vi "写入内置参数.vi"(7 "量程参数读取":T3 {"阈值（高->低）" format="%#.6g"; "阈值（低->高）" format="%#.6g"; "下限" format="%#.6g"; "上限" format="%#.6g"}, 8 "error in (no error)":errorcluster, 9 "float":T2 {"偏心轮校准参数" format="%#.6g"}, 10 "外设配置":T1 {"是否存在液位检测板" items=["否", "是"]; "阀数量" items=["9通"=9, "12通"=12]; "泵类型" items=["TECAN", "润泽"]}, 11 "MB session in":refnum<class "MB_Master.lvclass">) -> (0 "error out":errorcluster, 3 "MB session out":refnum<class "MB_Master.lvclass">)   [LabVIEW 2016, in "斯坦道CODMn新电路板.lvlib"]
uses:
  <vilib>/Plasmionique/MB Master/MB_Master/MB_Master.lvclass
  <vilib>/Plasmionique/MB Master/MB_Master_Serial/MB_Master_Serial.lvclass
  D:/Program Files (x86)/National Instruments/LabVIEW 2016/vi.lib/Plasmionique/MB Master/MB_Master/MB_Master.lvclass
  <vilib>/Plasmionique/MB Master/MB Master.lvlib
panel:
  in  "VISA Resource":refnum<visa-resource-name>
  in  "引用选择":enum16{"MB引用", "自建引用"}(ring)
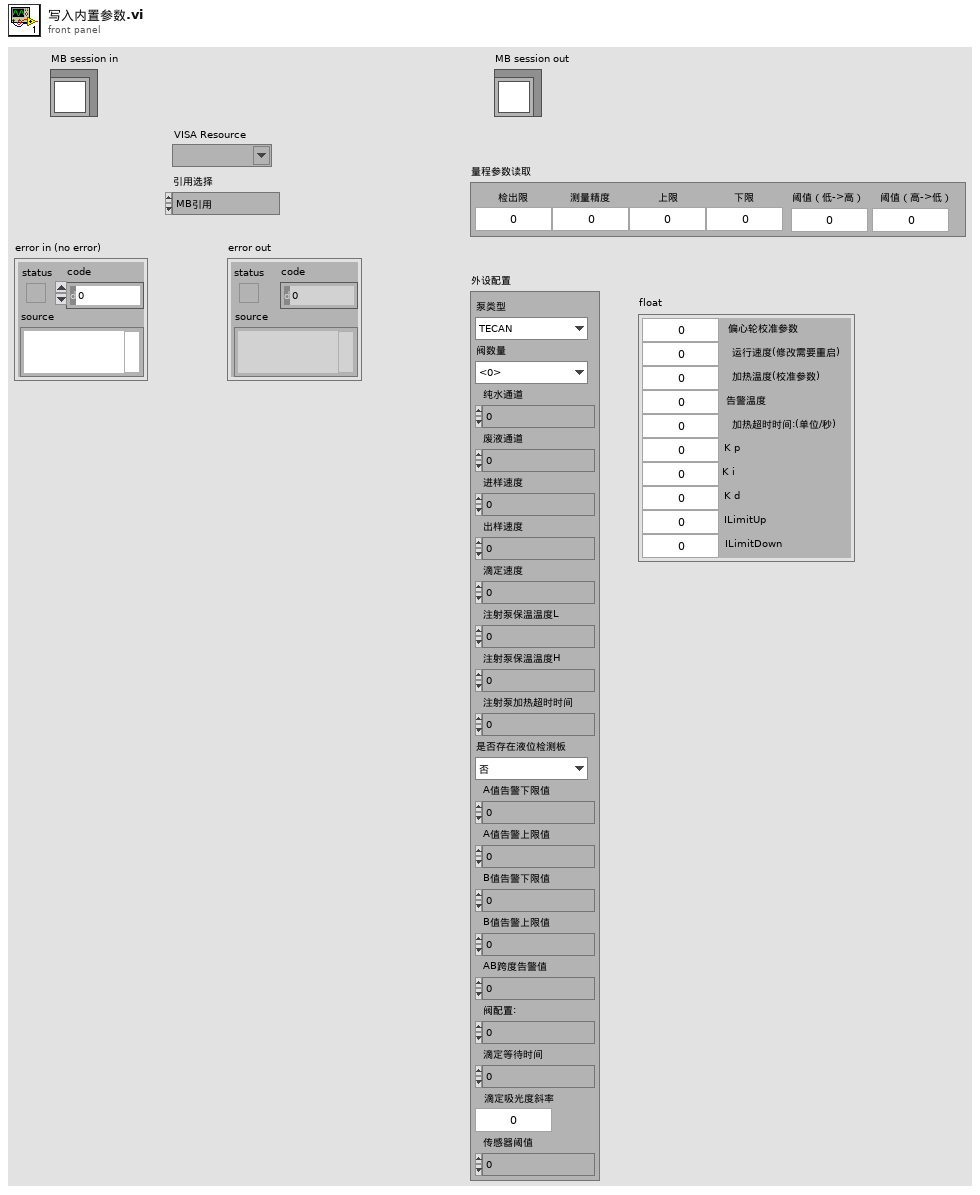
[diagram p1: front panel]
types:
  T1 = cluster{"泵类型":u8, "阀数量":u8, "纯水通道":u16, "废液通道":u8, "进样速度":u16, "出样速度":u16, "滴定速度":u16, "注射泵保温温度L":u8, "注射泵保温温度H":u8, "注射泵加热超时时间":u16, "是否存在液位检测板":u16, "A值告警下限值":u16, "A值告警上限值":u16, "B值告警下限值":u16, "B值告警上限值":u16, "AB跨度告警值":u16, "阀配置:":u8, "滴定等待时间":u16, "滴定吸光度斜率":dbl, "传感器阈值":u16}
  T2 = cluster{"偏心轮校准参数":dbl, "运行速度(修改需要重启)":u16, "加热温度(校准参数) ":dbl, "告警温度":dbl, "加热超时时间:(单位/秒)":dbl, "K p":dbl, "K i":dbl, "K d":dbl, "ILimitUp":dbl, "ILimitDown":dbl}
  T3 = cluster{"检出限":dbl, "测量精度":dbl, "上限":dbl, "下限":dbl, "阈值（低->高）":dbl, "阈值（高->低）":dbl}
  T4 = cluster{"baud rate (bps)":u32, "stop bits":u16, "parity":u16, "flow control":u16, "timeout":u32, "retries":i32}
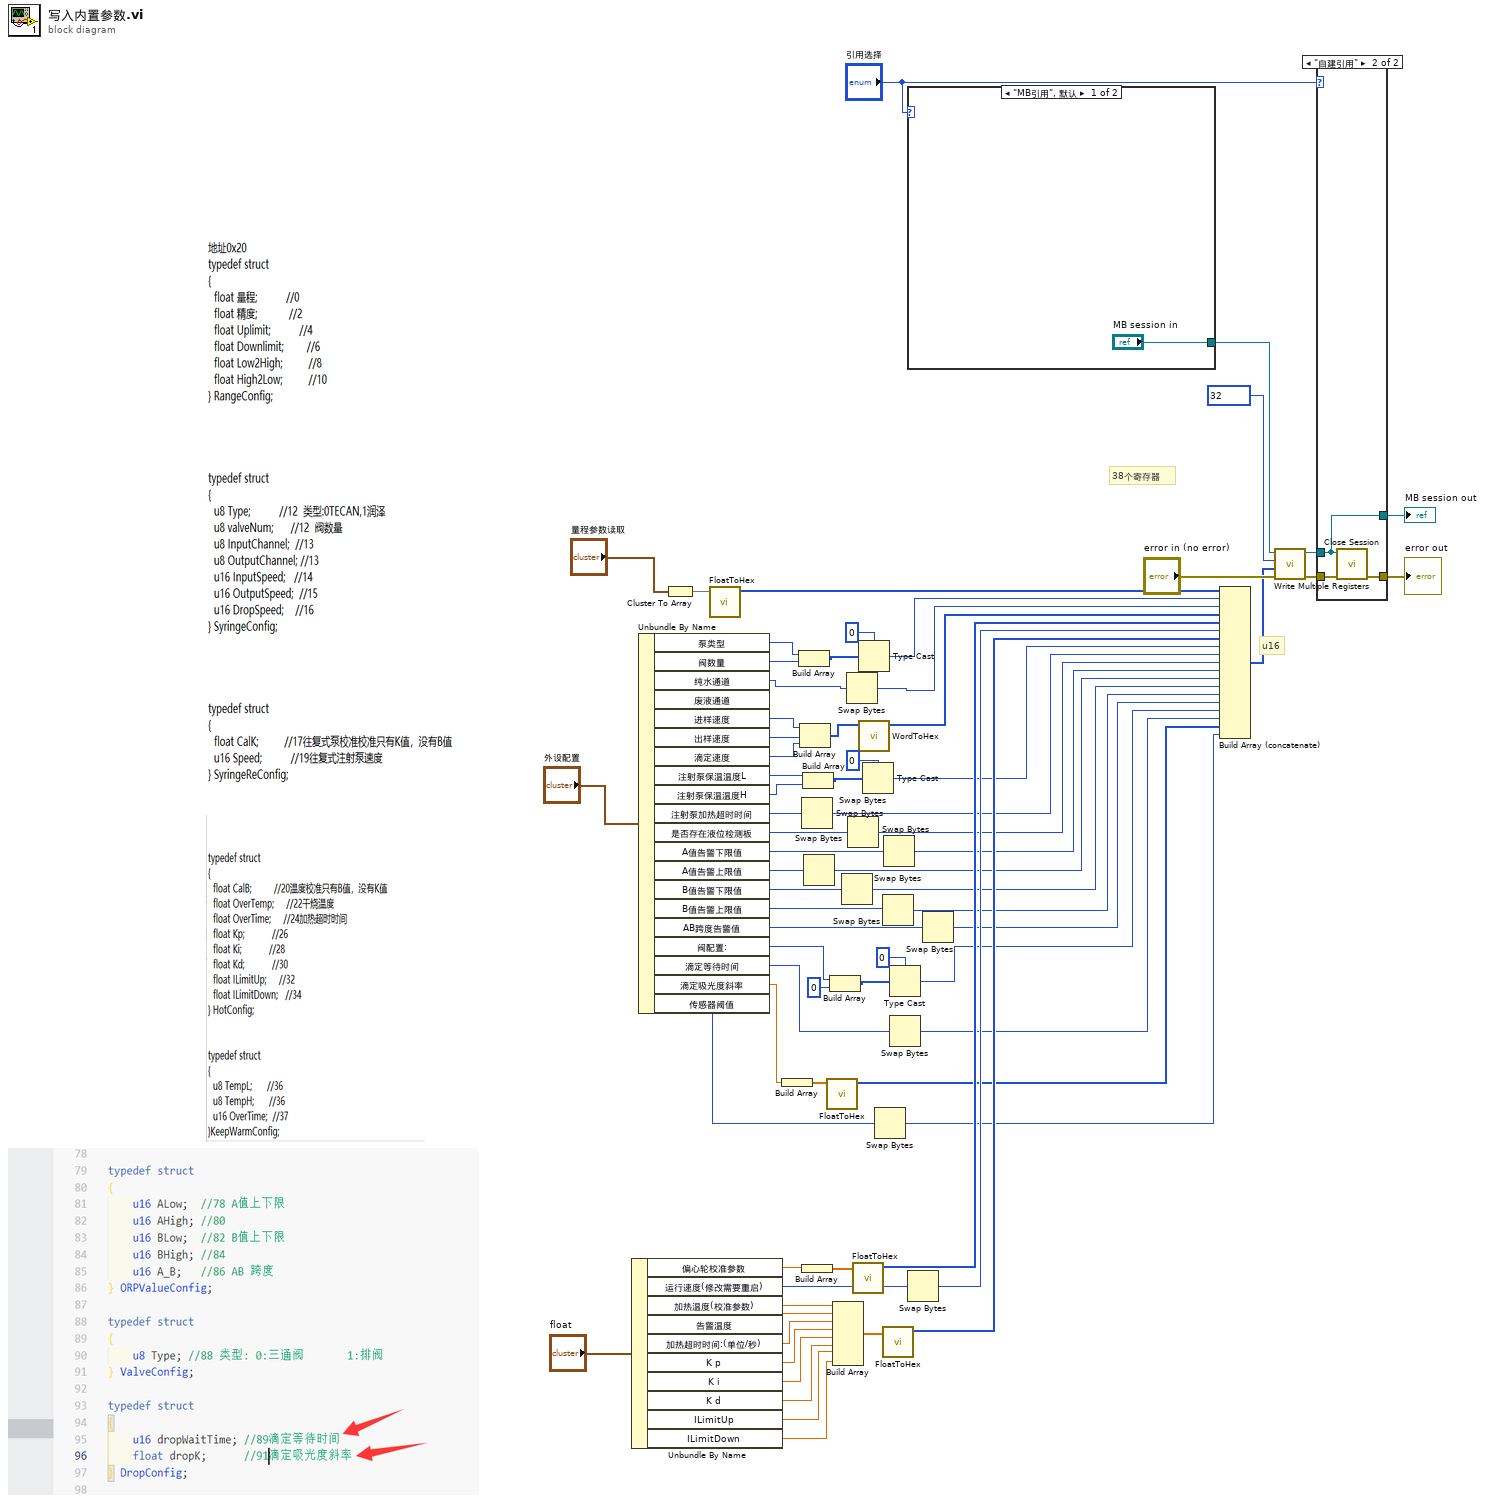
[diagram p0: block diagram]
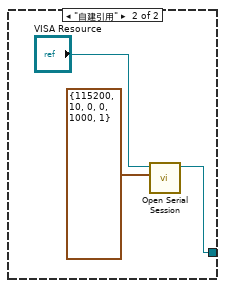
[diagram p3: hidden frame]
diagram:
  # "38个寄存器"
  # "u16"
  n1 = Unbundle By Name("float") -> ("偏心轮校准参数"=w55:dbl, "运行速度(修改需要重启)"=w32:u16, "加热温度(校准参数)"=w52:dbl, "告警温度"=w51:dbl, "加热超时时间:(单位/秒)"=w50:dbl, "K p"=w49:dbl, "K i"=w48:dbl, "K d"=w47:dbl, "ILimitUp"=w46:dbl, "ILimitDown"=w45:dbl)
  n2 = Unbundle By Name("外设配置") -> ("泵类型"=w62:u8, "阀数量"=w61:u8, "纯水通道"=w4:u16, "进样速度"=w38:u16, "出样速度"=w37:u16, "滴定速度"=w36:u16, "注射泵保温温度L"=w41:u8, "注射泵保温温度H"=w40:u8, "注射泵加热超时时间"=w39:u16, "是否存在液位检测板"=w27:u16, "A值告警下限值"=w25:u16, "A值告警上限值"=w24:u16, "B值告警下限值"=w23:u16, "B值告警上限值"=w22:u16, "AB跨度告警值"=w21:u16, "阀配置:"=w13:u8, "滴定等待时间"=w10:u16, "滴定吸光度斜率"=w8:dbl, "传感器阈值"=w2:u16)  [unwired: 1 out]
  n3 = Cluster To Array(cluster="量程参数读取") -> (array=w64:dbl[])
  n4 = call "FloatToHex.vi"("浮点数"=w64) -> ("DCBA整形输出"=w63:u16[])  [unwired: 10 in]
  n5 = Build Array(w8) -> (w7:dbl[])
  n6 = Build Array(w62, w61) -> (w58:u8[])
  n7 = Build Array(w38, w37, w36) -> (w35:u16[])
  n8 = Swap Bytes(anything=w39) -> (byte swapped=w28:u16)
  n9 = Build Array(w55) -> (w54:dbl[])
  n10 = Build Array(w41, w40) -> (w43:u8[])
  n11 = Swap Bytes(anything=w24) -> (byte swapped=w19:u16)
  n12 = call "FloatToHex.vi"("浮点数"=w7) -> ("DCBA整形输出"=w6:u16[])  [unwired: 10 in]
  n13 = Build Array(w13, u8 0 ("元素")) -> (w14:u8[])
  n14 = Build Array(w52, w51, w50, w49, w48, w47, w46, w45) -> (w44:dbl[])
  n15 = Swap Bytes(anything=w23) -> (byte swapped=w18:u16)
  n16 = Swap Bytes(anything=w4) -> (byte swapped=w3:u16)
  n17 = Swap Bytes(anything=w27) -> (byte swapped=w26:u16)
  n18 = call "FloatToHex.vi"("浮点数"=w54) -> ("DCBA整形输出"=w33:u16[])  [unwired: 10 in]
  n19 = Type Cast(type=u16 0, x=w58) -> (*(type *) &x=w56:u16)
  n20 = call "WordToHex.vi"("WORD"=w35) -> ("数组"=w34:u16[])  [unwired: 10 in]
  n21 = Type Cast(type=u16 0, x=w43) -> (*(type *) &x=w29:u16)
  n22 = Swap Bytes(anything=w2) -> (byte swapped=w1:u16)
  n23 = Swap Bytes(anything=w22) -> (byte swapped=w17:u16)
  n24 = call "FloatToHex.vi"("浮点数"=w44) -> ("DCBA整形输出"=w30:u16[])  [unwired: 10 in]
  n25 = Swap Bytes(anything=w25) -> (byte swapped=w20:u16)
  n26 = Type Cast(type=u16 0, x=w14) -> (*(type *) &x=w12:u16)
  n27 = Swap Bytes(anything=w10) -> (byte swapped=w9:u16)
  n28 = case shown="\"MB引用\", 默认" "引用选择" {
    tunnel: ["MB session in" w76] -> w70
    frame "MB引用", Default {
    }
    frame "自建引用" {
      n29 = call <vilib>:"Open Serial Session.vi"("Serial Config"=T4 {"baud rate (bps)"=115200, "stop bits"=10, "parity"=0, "flow control"=0, "timeout"=1000, "retries"=1}, "VISA Resource"="VISA Resource") -> ("MB_Serial session"=w76:refnum<class "MB_Master_Serial.lvclass">)  [unwired: 8 in, 1 out]
    }
  }
  n30 = Swap Bytes(anything=w32) -> (byte swapped=w31:u16)
  n31 = Swap Bytes(anything=w21) -> (byte swapped=w16:u16)
  n32 = Build Array (concatenate)(w63, w56, w3, w34, w33, w31, w30, w29, w28, w26, w20, w19, w18, w17, w16, w12, w9, w6, w1) -> (w57:u16[])
  n33 = call <vilib>:"Write Multiple Registers.vi"("error in (no error)"="error in (no error)", "values"=w57, "starting address"=u16 32, "MB session in"=w70) -> ("error out"=w67:errorcluster, "MB session out"=w69:refnum<class "MB_Master.lvclass">)  [unwired: 6 in]
  n34 = case shown="\"自建引用\"" "引用选择" {
    tunnel: w69 -> [w77 w79]
    tunnel: w67 -> [w78 w81]
    tunnel: [w78 w80] -> w66
    tunnel: [w77 w79] -> w65
    frame "MB引用", Default {
    }
    frame "自建引用" {
      n35 = call-dynamic "Close Session.vi"("error in (no error)"=w81, "MB session in"=w79) -> ("error out"=w80:errorcluster)  [unwired: 9 in]
    }
  }
  "MB session out" <- w65
  "error out" <- w66
